vi "Write Cycle running.vi"(10 "Cycle running":bool, 11 "Temperature Control in":refnum<class "Temperature Control.lvclass">) -> (3 "Temperature Control out":refnum<class "Temperature Control.lvclass">)   [LabVIEW 2020, in "Temperature Control.lvclass"]
uses:
  Temperature Control.lvclass
  Temperature Control.lvclass/Temperature Control.ctl
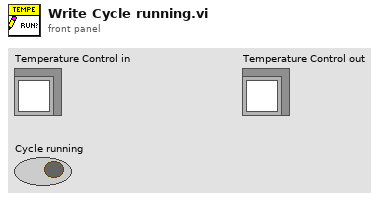
[diagram p1: front panel]
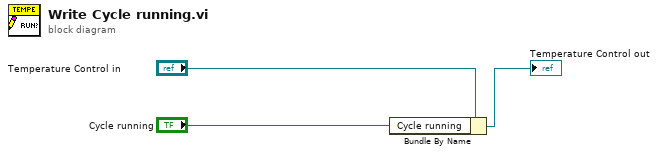
[diagram p0: block diagram]
diagram:
  n1 = Bundle By Name(cluster="Temperature Control in", "Cycle running"="Cycle running") -> (→"Temperature Control out":refnum<class "Temperature Control.lvclass">)
